vi "moreSamplesToPlayback_old.vi"(8 "bufferSize":i32, 11 "Device":i32) -> (0 "currentSampleCycle":i32, 3 "ReadyForMore":bool)   [LabVIEW 2011]
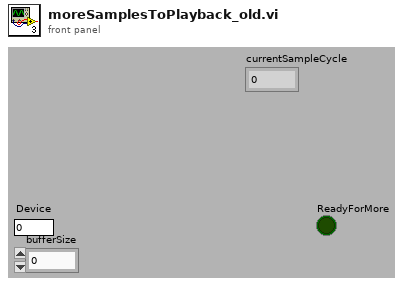
[diagram p1: front panel]
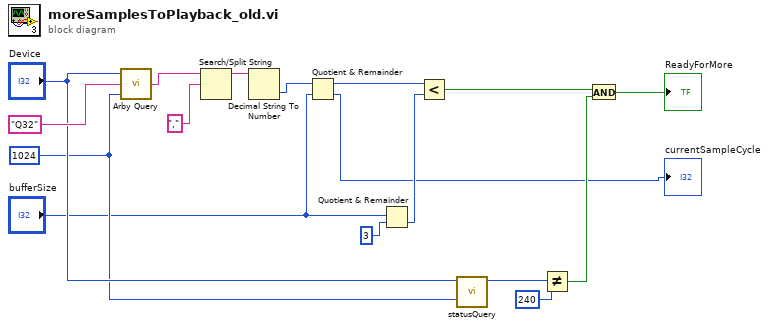
[diagram p0: block diagram]
diagram:
  w8 = 1024 ("Reply size")
  n1 = call "Arby Query.vi"("Reply size"=w8, "Query"="Q32", "Device"="Device") -> ("Reply"=w10:string)  [unwired: 2 out]
  n2 = Search/Split String(string=w10, search string/char (-)=",") -> (substring before match=w15:string)  [unwired: 1 in, 2 out]
  n3 = Decimal String To Number(string=w15) -> (number=w13:i32)  [unwired: 2 in, 1 out]
  n4 = Quotient & Remainder(x=w13, y="bufferSize") -> (x-y*floor(x/y)=w11:i32, floor(x/y)=→"currentSampleCycle":i32)
  n5 = Quotient & Remainder(x="bufferSize", y=3) -> (floor(x/y)=w12:i32)  [unwired: 1 out]
  n6 = Less?(x=w11, y=w12) -> (x < y?=w5:bool)
  n7 = call "statusQuery.vi"("Reply size"=w8, "Device ID"="Device") -> ("statusCode"=w7:i32)  [unwired: 8 in, 1 out]
  n8 = Not Equal?(x=w7, y=240) -> (x != y?=w4:bool)
  n9 = And(x=w5, y=w4) -> (x .and. y?=→"ReadyForMore":bool)
